vi "Dynamixel Single Function Sub.vi"(6 "data":u32, 7 "Function":T1, 8 "error In":errorcluster, 9 "Model Number":u32, 10 "dynamixel_id":u8=1, 11 "port_num":i32) -> (0 "error out":errorcluster, 1 "Value returned":i32)   [LabVIEW 2022 SP3]
uses:
  Dynamixel Commands.ctl
  Dynamixel VI type.ctl
  Dynamixel Global.vi
  Library/dxl.lvlib
panel:
  out "Array":string[](array[string])
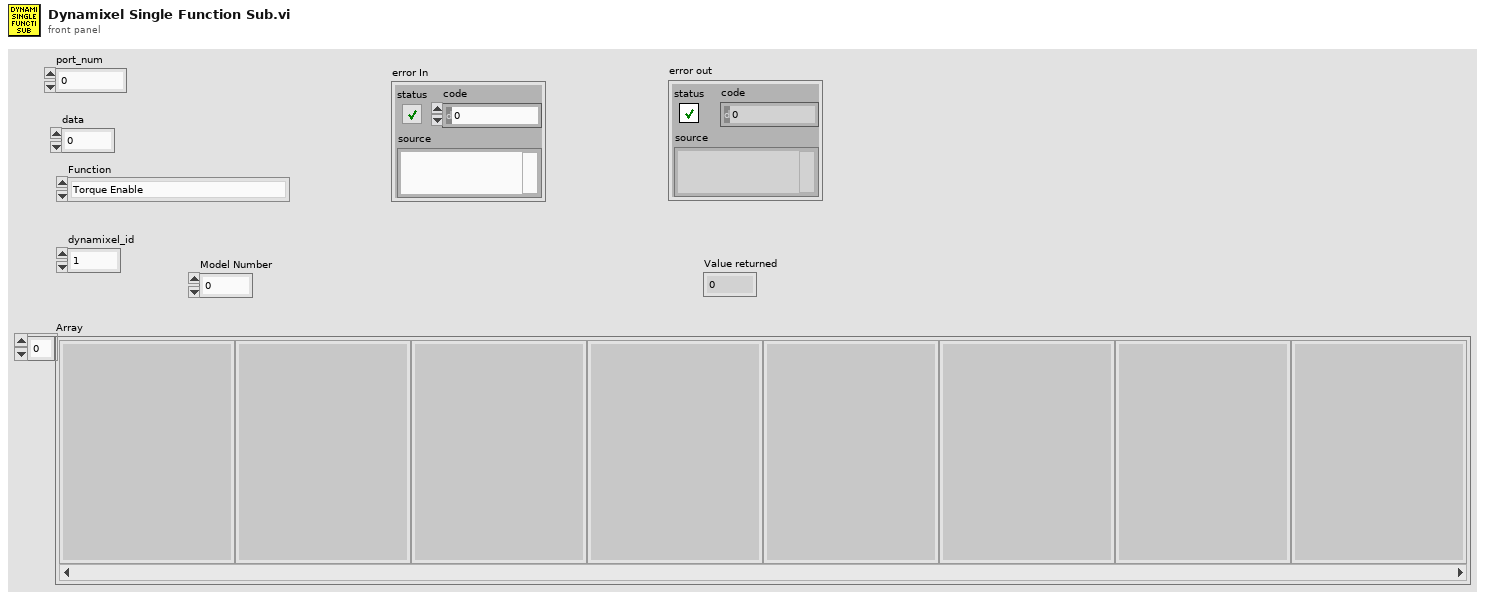
[diagram p1: front panel]
types:
  T1 = typedef "Dynamixel Commands.ctl" = enum16{"Torque Enable", "Present Position", "Threshold", "Max Position Limit", "Acceleration Profile", "Velocity Profile", "Goal Position", "Position Proportional Gain", "Position Integral Gain", "Position Differential Gain ", "Shutdown", "Write Operating Mode", "Read Operating Mode"}
  T2 = typedef "Dynamixel VI type.ctl" = enum16{"Write 2 Byte", "Read 4 Byte", "Write  4 Byte", "Read 1 Byte", "Write 1 Byte"}
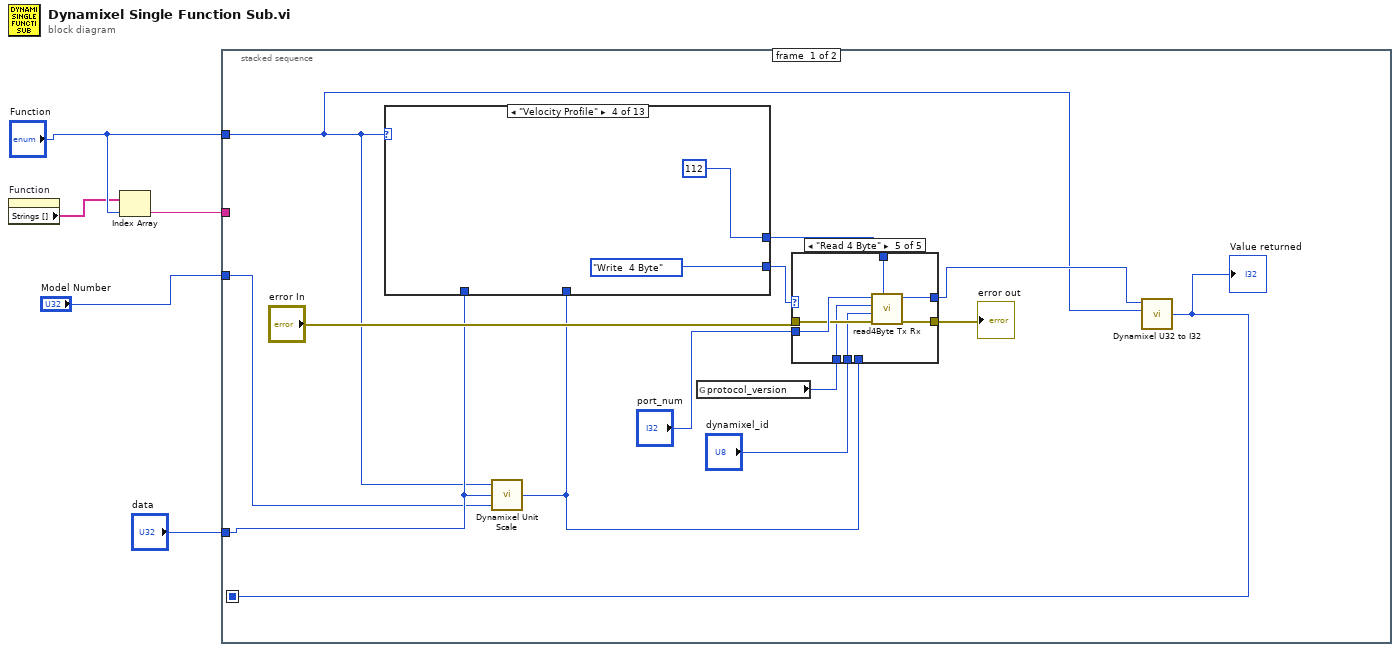
[diagram p0: block diagram]
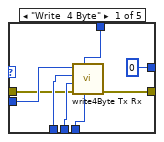
[diagram p2: hidden frame]
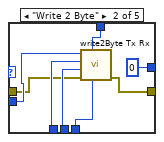
[diagram p3: hidden frame]
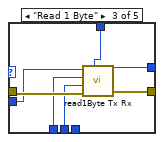
[diagram p4: hidden frame]
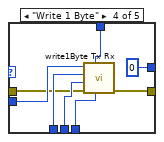
[diagram p5: hidden frame]
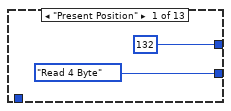
[diagram p6: hidden frame]
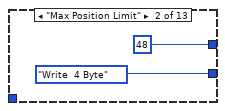
[diagram p7: hidden frame]
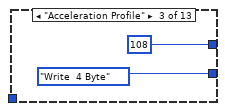
[diagram p8: hidden frame]
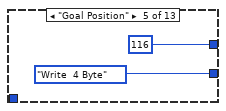
[diagram p9: hidden frame]
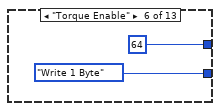
[diagram p10: hidden frame]
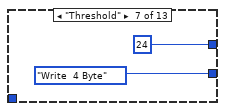
[diagram p11: hidden frame]
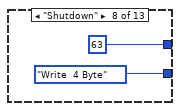
[diagram p12: hidden frame]
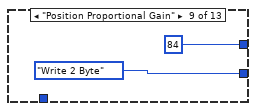
[diagram p13: hidden frame]
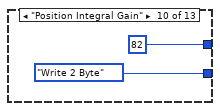
[diagram p14: hidden frame]
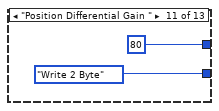
[diagram p15: hidden frame]
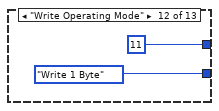
[diagram p16: hidden frame]
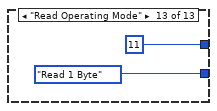
[diagram p17: hidden frame]
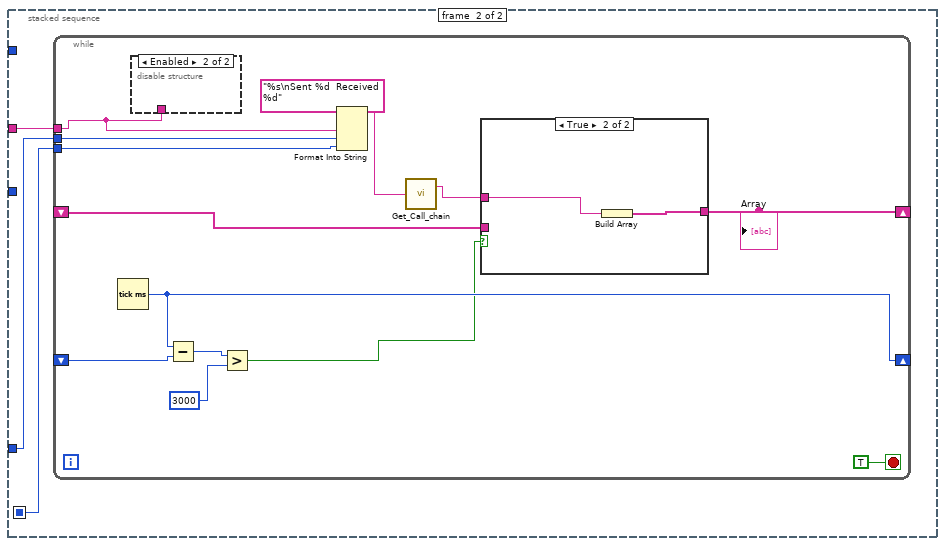
[diagram p18: hidden frame]
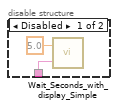
[diagram p19: hidden frame]
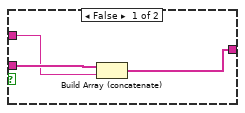
[diagram p20: hidden frame]
diagram:
  n1 = property on="Function" class="Enum (strict)"() -> ("Strings []"=w4:string[])  [unwired: 2 in, 2 out]
  n2 = Index Array(array=w4, index="Function") -> (element=w3:string)
  n3 = stacked-sequence {
    seq-local: [w6 _] -> [_ w83]
    tunnel: "Function" -> [w7 _]
    tunnel: w3 -> [_ w85]
    tunnel: "data" -> [w11 w84]
    tunnel: "Model Number" -> [w9 _]
    frame #0 {
      n4 = call "Dynamixel Unit Scale.vi"("Model Number"=w9, "Data in"=w11, "Function"=w7) -> ("Data out"=w10:u32)  [unwired: 2 in]
      n5 = case shown="\"Velocity Profile\"" w7 {
        tunnel: [u16 132 ("ADDR_PRO_\nPRESENT_POSITION") u16 48 ("ADDR_PRO_\nPRESENT_POSITION") u16 108 ("ADDR_PRO_\nPRESENT_POSITION") u16 112 ("ADDR_PRO_\nPRESENT_POSITION") u16 116 ("ADDR_PRO_\nPRESENT_POSITION") u16 64 ("ADDR_PRO_\nPRESENT_POSITION") u16 24 ("ADDR_PRO_\nPRESENT_POSITION") u16 63 ("ADDR_PRO_\nPRESENT_POSITION") u16 84 ("ADDR_PRO_\nPRESENT_POSITION") u16 82 ("ADDR_PRO_\nPRESENT_POSITION") u16 80 ("ADDR_PRO_\nPRESENT_POSITION") u16 11 ("ADDR_PRO_\nPRESENT_POSITION") u16 11 ("ADDR_PRO_\nPRESENT_POSITION")] -> w16
        tunnel: [Dynamixel_VI_type."Read 4 Byte" Dynamixel_VI_type."Write  4 Byte" Dynamixel_VI_type."Write  4 Byte" Dynamixel_VI_type."Write  4 Byte" Dynamixel_VI_type."Write  4 Byte" Dynamixel_VI_type."Write 1 Byte" Dynamixel_VI_type."Write  4 Byte" Dynamixel_VI_type."Write  4 Byte" Dynamixel_VI_type."Write 2 Byte" Dynamixel_VI_type."Write 2 Byte" Dynamixel_VI_type."Write 2 Byte" Dynamixel_VI_type."Write 1 Byte" Dynamixel_VI_type."Read 1 Byte"] -> w15
        tunnel: w10 -> [_ _ _ _ _ _ _ _ _ _ _ _ _]
        tunnel: w11 -> [_ _ _ _ _ _ _ _ _ _ _ _ _]
        frame "Present Position" {
        }
        frame "Max Position Limit" {
        }
        frame "Acceleration Profile" {
        }
        frame "Velocity Profile" {
        }
        frame "Goal Position" {
        }
        frame "Torque Enable" {
        }
        frame "Threshold" {
        }
        frame "Shutdown" {
        }
        frame "Position Proportional Gain" {
        }
        frame "Position Integral Gain" {
        }
        frame "Position Differential Gain " {
        }
        frame "Write Operating Mode" {
        }
        frame "Read Operating Mode" {
        }
      }
      n6 = global read "Dynamixel Global.vi" "protocol_version"() -> (w12:i32)
      n7 = case shown="\"Read 4 Byte\"" w15 {
        tunnel: "port_num" -> [w25 w32 w36 w46 w56]
        tunnel: "error In" -> [w22 w31 w39 w42 w55]
        tunnel: [w21 w28 w40 w43 w54] -> w13
        tunnel: w12 -> [w23 w34 w37 w47 w53]
        tunnel: "dynamixel_id" -> [w24 w33 w38 w48 w52]
        tunnel: w16 -> [w26 w30 w35 w45 w51]
        tunnel: [u32 0 ("function return") u32 0 ("function return") w41 u32 0 ("function return") w50] -> w8
        tunnel: w10 -> [w20 w29 _ w49 _]
        frame "Write  4 Byte" {
          n8 = call "write4Byte Tx Rx.vi"("data"=w20, "address"=w26, "error in (no error)"=w22, "id"=w24, "protocol_version"=w23, "port_num"=w25) -> ("error out"=w21:errorcluster)  [unwired: 5 in]
        }
        frame "Write 2 Byte" {
          n9 = call "write2Byte Tx Rx.vi"("data"=w29, "address"=w30, "error in (no error)"=w31, "id"=w33, "protocol_version"=w34, "port_num"=w32) -> ("error out"=w28:errorcluster)  [unwired: 5 in]
        }
        frame "Read 1 Byte" {
          n10 = call "read1Byte Tx Rx.vi"("address"=w35, "error in (no error)"=w39, "id"=w38, "protocol_version"=w37, "port_num"=w36) -> ("error out"=w40:errorcluster, "function return"=w41:u8)  [unwired: 5 in]
        }
        frame "Write 1 Byte" {
          n11 = call "write1Byte Tx Rx.vi"("data"=w49, "address"=w45, "error in (no error)"=w42, "id"=w48, "protocol_version"=w47, "port_num"=w46) -> ("error out"=w43:errorcluster)  [unwired: 5 in]
        }
        frame "Read 4 Byte" {
          n12 = call "read4Byte Tx Rx.vi"("address"=w51, "error in (no error)"=w55, "id"=w52, "protocol_version"=w53, "port_num"=w56) -> ("error out"=w54:errorcluster, "function return"=w50:u32)  [unwired: 5 in]
        }
      }
      "error out" <- w13
      n13 = call "Dynamixel U32 to I32.vi"("U32 In"=w8, "Function"=w7) -> ("I32 Out"=w6:i32)  [unwired: 3 in]
      "Value returned" <- w6
    }
    frame #1 {
      n14 = while {
        tunnel: w85 -> [w88]
        shift-right: [w99] -> _
        shift-left: _ -> [w98]
        shift-right: [w94] -> _
        shift-left: _ -> [w92]
        tunnel: w84 -> [w90]
        tunnel: w83 -> [w86]
        stop <- TRUE stop-if-true
        n15 = Tick Count (ms)() -> (millisecond timer value=w99:u32)
        n16 = disable-structure shown="Enabled" {
          disable-tunnel: w88 -> [w100 _]
          frame Disabled {
            n17 = call "Wait_Seconds_with_display_Simple.vi"("Message"=w100, "Seconds to wait"=5.0) -> ()  [unwired: 1 in, 1 out]
          }
          frame Enabled {
          }
        }
        n18 = Subtract(x=w99, y=w98) -> (x-y=w97:u32)
        n19 = Greater?(x=w97, y=u32 3000) -> (0:w95:bool)
        n20 = Format Into String(format string="%s\nSent %d  Received %d", w88, w90, w86) -> (resulting string=w87:string)  [unwired: 2 in, 1 out]
        n21 = call "Get_Call_chain.vi"("Message"=w87) -> ("Output String"=w93:string)  [unwired: 1 out]
        n22 = case shown="True" w95 {
          tunnel: [w103 w106] -> w94
          tunnel: w93 -> [w102 w105]
          tunnel: w92 -> [w104 _]
          frame False {
            n23 = Build Array (concatenate)(w104, w102) -> (w103:string[])
          }
          frame True {
            n24 = Build Array(w105) -> (w106:string[])
          }
        }
        "Array" <- w94
      }
    }
  }
